vi "NavbalLabVIEW(15-5-28.vi"() -> ()   [LabVIEW 2012] (continued)
                }
              }
            }
          }
          "Phase Corner" <- w3618
          n781 = case "Pick out Mag, Phase, and Weight locations from Excel File" shown="True" "Slct Strt Pt" {
            tunnel: "Marker Listbox" -> [_ w3714]
            tunnel: w3337 -> [_ w3728]
            tunnel: w3329 -> [_ w3711]
            frame False {
            }
            frame True {
              n782 = property on="Marker Listbox" class="MCListbox (strict)"() -> ("ItemNames"=w3713:string[][])  [unwired: 2 in, 2 out]
              n783 = case shown="\"Stbd Side\"" w3711 {
                tunnel: [w3768 w3770] -> w3719
                tunnel: [4 ("y") 5 ("x")] -> w3708
                frame "Port Side", Default {
                  n784 = local read "#Stbd Accels"() -> (w3768:i32)
                }
                frame "Stbd Side" {
                  n785 = local read "#Port Accels"() -> (w3770:i32)
                }
              }
              n786 = Multiply(x=w3714, y=2) -> (x*y=w3726:i32)
              n787 = Increment(x=w3726) -> (x+1=w3724:i32)
              n788 = Index Array(array=w3713, index (row)=w3714, index (col)=0 ("disabled index (col)")) -> (element=→"Indicate Ref":string)
              n789 = call <vilib>:"New Report.vi"("report type"=T11."Excel", "template (empty)"=w3728) -> ("report out"=w3734:refnum<class "NI_report.lvclass">, "error out"=w3735:errorcluster)  [unwired: 12 in]
              n790 = Bundle("y"=12, w3724) -> (w3731:cluster{"y":i32, i32})  [unwired: 1 in]
              n791 = call <vilib>:"Excel Get Worksheet.vi"("report in"=w3734, "worksheet index (0)"=w3708, "error in (no error)"=w3735) -> ("report out"=w3737:refnum<class "NI_report.lvclass">, "error out"=w3738:errorcluster)  [unwired: 11 out]
              n792 = local read "#Corner Accels"() -> (w3718:i32)
              n793 = Increment(x=w3724) -> (x+1=w3725:i32)
              n794 = local read "#Corner Accels"() -> (w3709:i32)
              n795 = Add(x=w3718, y=w3719) -> (x+y=w3720:i32)
              n796 = Add(x=12, y=w3720) -> (x+y=w3722:i32)
              n797 = Decrement(x=w3722) -> (x-1=w3717:i32)
              n798 = Bundle(w3717, w3725) -> (w3730:cluster{i32, i32})  [unwired: 1 in]
              n799 = call-poly <vilib>:"Excel Get Data.vi"("report in"=w3737, "data type"=string[][] [], "start (-1, -1)"=w3731, "end (-1, -1)"=w3730, "error in (no error)"=w3738) -> ("data"=w3729:string[][], "error out"=w3723:errorcluster)  [unwired: 9 out]
              n800 = call <vilib>:"General Error Handler.vi"("error in (no error)"=w3723) -> ()  [unwired: 2 in, 13 out]
              n801 = Fract/Exp String To Number(string=w3729) -> (number=w3710:dbl[][])  [unwired: 3 in, 1 out]
              n802 = case shown="\"Port Side\", Default" w3711 {
                tunnel: w3710 -> [w3752 w3766]
                tunnel: [w3744 w3757] -> w3712
                tunnel: w3709 -> [w3741 w3756]
                frame "Port Side", Default {
                  n803 = Initialize Array(0.0 ("element"), w3741, 2 ("dimension size")) -> (w3749:dbl[][])
                  n804 = Insert Into Array(array=w3752, index (row)=0, new element=w3749) -> (w3748:dbl[][])  [unwired: 1 in]
                  n805 = Multiply(x=2, y=w3741) -> (x*y=w3740:i32)
                  n806 = local read "#Stbd Accels"() -> (w3739:i32)
                  n807 = Initialize Array(0.0 ("element"), w3739, 2 ("dimension size")) -> (w3745:dbl[][])
                  n808 = Insert Into Array(array=w3748, index (row)=w3740, new element=w3745) -> (w3744:dbl[][])  [unwired: 1 in]
                }
                frame "Stbd Side" {
                  n809 = local read "#Stbd Accels"() -> (w3753:i32)
                  n810 = Initialize Array(0.0 ("element"), w3756, 2 ("dimension size")) -> (w3763:dbl[][])
                  n811 = Insert Into Array(array=w3766, index (row)=w3756, new element=w3763) -> (w3762:dbl[][])  [unwired: 1 in]
                  n812 = Multiply(x=2, y=w3756) -> (x*y=w3754:i32)
                  n813 = Add(x=w3754, y=w3753) -> (x+y=w3761:i32)
                  n814 = Initialize Array(0.0 ("element"), w3753, 2 ("dimension size")) -> (w3758:dbl[][])
                  n815 = Insert Into Array(array=w3762, index (row)=w3761, new element=w3758) -> (w3757:dbl[][])  [unwired: 1 in]
                }
              }
              "Ref Pt Plot" <- w3712
            }
          }
          n816 = case shown="True" "Refresh Plot Listbox" {
            tunnel: w3337 -> [_ w3779]
            frame False {
            }
            frame True {
              n817 = local read "Port/Starboard"() -> (w3782:enum32{"Port Side", "Stbd Side"})
              n818 = case shown="\"Port Side\", Default" w3782 {
                tunnel: ["Data-Port" "Data-Stbd"] -> w3781
                frame "Port Side", Default {
                }
                frame "Stbd Side" {
                }
              }
              n819 = call <vilib>:"New Report.vi"("report type"=T11."Excel", "template (empty)"=w3779) -> ("report out"=w3785:refnum<class "NI_report.lvclass">, "error out"=w3784:errorcluster)  [unwired: 12 in]
              n820 = call <vilib>:"Excel Get Worksheet.vi"("report in"=w3785, "error in (no error)"=w3784, "name (\"\")"=w3781) -> ("report out"=w3798:refnum<class "NI_report.lvclass">, "error out"=w3797:errorcluster)  [unwired: 1 in, 10 out]
              n821 = Increment(x="# Runs") -> (x+1=w3786:dbl)
              n822 = Multiply(x=w3786, y=2) -> (x*y=w3788:dbl)
              n823 = Bundle("row"=2, w3788) -> (w3787:cluster{"row":i32, dbl})  [unwired: 1 in]
              n824 = call-poly <vilib>:"Excel Get Data.vi"("report in"=w3798, "data type"=string[][] [], "start (-1, -1)"=cluster{"row":i32, "column":i32} {"row"=0, "column"=1}, "end (-1, -1)"=w3787, "error in (no error)"=w3797) -> ("data"=w3792:string[][])  [unwired: 10 out]
              n825 = Transpose 2D Array(2D array=w3792) -> (transposed array=w3795:string[][])
              n826 = local read "Predicted Phase"() -> (w3775:dbl[])
              n827 = Index Array(array=w3795, index (col)=0 ("disabled index (col)")) -> (element=w3794:string[])  [unwired: 1 in]
              n828 = Decimate 1D Array(w3794) -> (w3791:string[])  [unwired: 1 out]
              n829 = Array Size(array=w3791) -> (size(s)=w3793:i32)
              n830 = Reshape Array(w3791, w3793, 1 ("dimension size")) -> (w3783:string[][])
              n831 = local read "Predicted Mag"() -> (w3776:dbl[])
              n832 = local read "Select Side to Analyze"() -> (w3771:enum32{"Starboard", "Port"})
              n833 = property on="Marker Listbox" class="MCListbox (strict)"("ItemNames"=w3783) -> ()  [unwired: 2 in, 2 out]
              n834 = local read "#Corner Accels"() -> (w3773:i32)
              n835 = Build Array(w3776, w3775) -> (w3777:dbl[][])
              n836 = Transpose 2D Array(2D array=w3777) -> (transposed array=w3774:dbl[][])
              n837 = case shown="\"Port\"" w3771 {
                tunnel: w3774 -> [w3815 w3829]
                tunnel: [w3806 w3821] -> w3772
                tunnel: w3773 -> [w3805 w3818]
                frame "Starboard", Default {
                  n838 = local read "#Stbd Accels"() -> (w3802:i32)
                  n839 = Initialize Array(0.0 ("element"), w3805, 2 ("dimension size")) -> (w3812:dbl[][])
                  n840 = Insert Into Array(array=w3815, index (row)=w3805, new element=w3812) -> (w3811:dbl[][])  [unwired: 1 in]
                  n841 = Multiply(x=2, y=w3805) -> (x*y=w3803:i32)
                  n842 = Add(x=w3803, y=w3802) -> (x+y=w3810:i32)
                  n843 = Initialize Array(0.0 ("element"), w3802, 2 ("dimension size")) -> (w3807:dbl[][])
                  n844 = Insert Into Array(array=w3811, index (row)=w3810, new element=w3807) -> (w3806:dbl[][])  [unwired: 1 in]
                }
                frame "Port" {
                  n845 = Initialize Array(0.0 ("element"), w3818, 2 ("dimension size")) -> (w3826:dbl[][])
                  n846 = Insert Into Array(array=w3829, index (row)=0, new element=w3826) -> (w3825:dbl[][])  [unwired: 1 in]
                  n847 = Multiply(x=2, y=w3818) -> (x*y=w3817:i32)
                  n848 = local read "#Stbd Accels"() -> (w3816:i32)
                  n849 = Initialize Array(0.0 ("element"), w3816, 2 ("dimension size")) -> (w3822:dbl[][])
                  n850 = Insert Into Array(array=w3825, index (row)=w3817, new element=w3822) -> (w3821:dbl[][])  [unwired: 1 in]
                }
              }
              "Pred plot" <- w3772
            }
          }
          n851 = Divide(x=159.0, y=w3556) -> (x/y=w3700:dbl)
          n852 = Divide(x=159.0, y=w3557) -> (x/y=w3685:dbl)
          n853 = Logarithm Base 10(1:w3700) -> (0:w3699:dbl)
          n854 = Divide(x=159.0, y=w3643) -> (x/y=w3658:dbl)
          n855 = Logarithm Base 10(1:w3685) -> (0:w3684:dbl)
          n856 = Divide(x=159.0, y=w3483) -> (x/y=w3509:dbl)
          n857 = Multiply(x=20.0, y=w3699) -> (x*y=w3698:dbl)
          n858 = Logarithm Base 10(1:w3658) -> (0:w3657:dbl)
          n859 = Multiply(x=20.0, y=w3684) -> (x*y=w3683:dbl)
          n860 = Logarithm Base 10(1:w3509) -> (0:w3508:dbl)
          n861 = Subtract(x=w3696, y=w3698) -> (x-y=w3692:dbl[][])
          "Magnitude AdB Stbd" <- w3692
          n862 = Multiply(x=20.0, y=w3657) -> (x*y=w3656:dbl)
          n863 = Subtract(x=w3681, y=w3683) -> (x-y=w3674:dbl[][])
          "Magnitude AdB Port" <- w3674
          n864 = Multiply(x=20.0, y=w3508) -> (x*y=w3507:dbl)
          n865 = Subtract(x=w3644, y=w3656) -> (x-y=w3642:dbl[][])
          "Magnitude AdB Corner" <- w3642
          n866 = Subtract(x=w3495, y=w3507) -> (x-y=w3494:dbl[][])
          "Magnitude AdB Corners-Port" <- w3494
          n867 = local read "Averaging"() -> (w3365:bool)
          n868 = for "Mils(8x)" {
            N: w3521 -> [_]
            tunnel: w3696 -> [w5013]
            tunnel: w3556 -> [w5009]
            tunnel: [w5008] -> w3639 mode=indexing
            tunnel: [w5007] -> w3697 mode=indexing
            i -> [w5010]
            n869 = Index Array(array=w5013, index (row)=w5010) -> (element=w5011:dbl[])  [unwired: 1 in]
            n870 = for {
              N: 8 -> [_]
              tunnel: w5011 -> [w5022]
              tunnel: w5009 -> [w5030]
              tunnel: [w5016] -> w5008 mode=indexing
              tunnel: [w5014] -> w5007 mode=indexing
              i -> [w5029]
              n871 = Add(x=w5029, y=1) -> (x+y=w5031:i32)
              n872 = Index Array(array=w5022, index=w5029) -> (element=w5023:dbl)
              n873 = Multiply(x=w5030, y=w5031) -> (x*y=w5014:dbl)
              n874 = Divide(x=159, y=w5014) -> (x/y=w5027:dbl)
              n875 = Logarithm Base 10(1:w5027) -> (0:w5026:dbl)
              n876 = Multiply(x=20.0, y=w5026) -> (x*y=w5024:dbl)
              n877 = Subtract(x=w5023, y=w5024) -> (x-y=w5017:dbl)
              n878 = Divide(x=w5017, y=20.0) -> (x/y=w5019:dbl)
              n879 = Power Of 10(x=w5019) -> (10^x=w5021:dbl)
              n880 = Multiply(x=w5021, y=0.0887) -> (x*y=w5015:dbl)
              n881 = Divide(x=w5015, y=w5014) -> (x/y=w5016:dbl)
            }
          }
          "Mils/sec Stbd" <- w3639
          "Freq Stbd" <- w3697
          n882 = for "Mils(8x)" {
            N: w3519 -> [_]
            tunnel: w3681 -> [w4905]
            tunnel: w3557 -> [w4901]
            tunnel: [w4900] -> w3619 mode=indexing
            tunnel: [w4899] -> w3682 mode=indexing
            i -> [w4902]
            n883 = Index Array(array=w4905, index (row)=w4902) -> (element=w4903:dbl[])  [unwired: 1 in]
            n884 = for {
              N: 8 -> [_]
              tunnel: w4903 -> [w4914]
              tunnel: w4901 -> [w4922]
              tunnel: [w4908] -> w4900 mode=indexing
              tunnel: [w4906] -> w4899 mode=indexing
              i -> [w4921]
              n885 = Add(x=w4921, y=1) -> (x+y=w4923:i32)
              n886 = Index Array(array=w4914, index=w4921) -> (element=w4915:dbl)
              n887 = Multiply(x=w4922, y=w4923) -> (x*y=w4906:dbl)
              n888 = Divide(x=159, y=w4906) -> (x/y=w4919:dbl)
              n889 = Logarithm Base 10(1:w4919) -> (0:w4918:dbl)
              n890 = Multiply(x=20.0, y=w4918) -> (x*y=w4916:dbl)
              n891 = Subtract(x=w4915, y=w4916) -> (x-y=w4909:dbl)
              n892 = Divide(x=w4909, y=20.0) -> (x/y=w4911:dbl)
              n893 = Power Of 10(x=w4911) -> (10^x=w4913:dbl)
              n894 = Multiply(x=w4913, y=0.0887) -> (x*y=w4907:dbl)
              n895 = Divide(x=w4907, y=w4906) -> (x/y=w4908:dbl)
            }
          }
          "Mils/sec Port" <- w3619
          "Freq Port" <- w3682
          n896 = Index Array(array=w3692, index (col)=0 ("disabled index (col)")) -> (element=w3693:dbl[])  [unwired: 1 in]
          n897 = local read "Averaging"() -> (w3358:bool)
          n898 = for "Mils(8x)" {
            N: w3571 -> [_]
            tunnel: w3644 -> [w4717]
            tunnel: w3643 -> [w4713]
            tunnel: [w4712] -> w3617 mode=indexing
            tunnel: [w4711] -> w3655 mode=indexing
            i -> [w4714]
            n899 = Index Array(array=w4717, index (row)=w4714) -> (element=w4715:dbl[])  [unwired: 1 in]
            n900 = for {
              N: 8 -> [_]
              tunnel: w4715 -> [w4726]
              tunnel: w4713 -> [w4734]
              tunnel: [w4720] -> w4712 mode=indexing
              tunnel: [w4718] -> w4711 mode=indexing
              i -> [w4733]
              n901 = Add(x=w4733, y=1) -> (x+y=w4735:i32)
              n902 = Index Array(array=w4726, index=w4733) -> (element=w4727:dbl)
              n903 = Multiply(x=w4734, y=w4735) -> (x*y=w4718:dbl)
              n904 = Divide(x=159, y=w4718) -> (x/y=w4731:dbl)
              n905 = Logarithm Base 10(1:w4731) -> (0:w4730:dbl)
              n906 = Multiply(x=20.0, y=w4730) -> (x*y=w4728:dbl)
              n907 = Subtract(x=w4727, y=w4728) -> (x-y=w4721:dbl)
              n908 = Divide(x=w4721, y=20.0) -> (x/y=w4723:dbl)
              n909 = Power Of 10(x=w4723) -> (10^x=w4725:dbl)
              n910 = Multiply(x=w4725, y=0.0887) -> (x*y=w4719:dbl)
              n911 = Divide(x=w4719, y=w4718) -> (x/y=w4720:dbl)
            }
          }
          "Mils/sec Corner" <- w3617
          "Freq Corner" <- w3655
          n912 = Index Array(array=w3674, index (col)=0 ("disabled index (col)")) -> (element=w3678:dbl[])  [unwired: 1 in]
          n913 = for "Mils(8x)" {
            N: w3481 -> [_]
            tunnel: w3495 -> [w4264]
            tunnel: w3483 -> [w4260]
            tunnel: [w4259] -> w3485 mode=indexing
            tunnel: [w4258] -> w3506 mode=indexing
            i -> [w4261]
            n914 = Index Array(array=w4264, index (row)=w4261) -> (element=w4262:dbl[])  [unwired: 1 in]
            n915 = for {
              N: 8 -> [_]
              tunnel: w4262 -> [w4273]
              tunnel: w4260 -> [w4281]
              tunnel: [w4267] -> w4259 mode=indexing
              tunnel: [w4265] -> w4258 mode=indexing
              i -> [w4280]
              n916 = Add(x=w4280, y=1) -> (x+y=w4282:i32)
              n917 = Index Array(array=w4273, index=w4280) -> (element=w4274:dbl)
              n918 = Multiply(x=w4281, y=w4282) -> (x*y=w4265:dbl)
              n919 = Divide(x=159, y=w4265) -> (x/y=w4278:dbl)
              n920 = Logarithm Base 10(1:w4278) -> (0:w4277:dbl)
              n921 = Multiply(x=20.0, y=w4277) -> (x*y=w4275:dbl)
              n922 = Subtract(x=w4274, y=w4275) -> (x-y=w4268:dbl)
              n923 = Divide(x=w4268, y=20.0) -> (x/y=w4270:dbl)
              n924 = Power Of 10(x=w4270) -> (10^x=w4272:dbl)
              n925 = Multiply(x=w4272, y=0.0887) -> (x*y=w4266:dbl)
              n926 = Divide(x=w4266, y=w4265) -> (x/y=w4267:dbl)
            }
          }
          "Mils/sec Corners-Port" <- w3485
          "Freq Corner Port" <- w3506
          n927 = local read "Averaging"() -> (w3356:bool)
          n928 = local read "Averaging"() -> (w3357:bool)
          n929 = Index Array(array=w3642, index (col)=0 ("disabled index (col)")) -> (element=w3652:dbl[])  [unwired: 1 in]
          n930 = Array Size(array=w3693) -> (size(s)=w3695:i32)
          n931 = Index Array(array=w3494, index (col)=0 ("disabled index (col)")) -> (element=w3503:dbl[])  [unwired: 1 in]
          n932 = Index Array(array=w3639, index (col)=0 ("index (row)")) -> (element=w3363:dbl[])  [unwired: 1 in]
          n933 = Index Array(array=w3558, index (col)=0 ("index")) -> (element=w3364:dbl[])  [unwired: 1 in]
          n934 = Index Array(array=w3692, index (col)=0 ("index (row)")) -> (element=w3361:dbl[])  [unwired: 1 in]
          n935 = Array Size(array=w3678) -> (size(s)=w3680:i32)
          n936 = Index Array(array=w3619, index (col)=0 ("index (row)")) -> (element=w3675:dbl[])  [unwired: 1 in]
          n937 = case shown="True" w3365 {
            tunnel: [w3879 w3880] -> w3362
            tunnel: w3364 -> [w3879 w3881]
            frame False {
            }
            frame True {
              n938 = call "Time Averaging3"("input signals"=w3881) -> ("time avg. signal"=w3880:dbl[])  [unwired: 15 in, 3 out]
            }
          }
          n939 = Index Array(array=w3415, index (col)=0 ("index")) -> (element=w3414:dbl[])  [unwired: 1 in]
          n940 = Index Array(array=w3674, index (col)=0 ("index (row)")) -> (element=w3673:dbl[])  [unwired: 1 in]
          n941 = Array Size(array=w3652) -> (size(s)=w3654:i32)
          n942 = for "Mils(1x)" {
            N: w3695 -> [_]
            tunnel: w3556 -> [w5002]
            tunnel: [w4997] -> w3360 mode=indexing
            tunnel: w3693 -> [w4996]
            i -> [w5006]
            n943 = Square(x=w5002) -> (x^2=w5000:dbl)
            n944 = Index Array(array=w4996, index #1=w5006) -> (element #1=w5005:dbl)  [unwired: 1 in, 1 out]
            n945 = Divide(x=0.028175, y=w5000) -> (x/y=w4998:dbl)
            n946 = Divide(x=w5005, y=20.0) -> (x/y=w5003:dbl)
            n947 = Power Of 10(x=w5003) -> (10^x=w4999:dbl)
            n948 = Multiply(x=w4999, y=w4998) -> (x*y=w4997:dbl)
          }
          "Mils(1x) Stbd" <- w3360
          n949 = case shown="True" w3358 {
            tunnel: w3414 -> [w3876 w3878]
            tunnel: [w3876 w3877] -> w3408
            frame False {
            }
            frame True {
              n950 = call "Time Averaging2"("input signals"=w3878) -> ("time avg. signal"=w3877:dbl[])  [unwired: 15 in, 3 out]
            }
          }
          n951 = Index Array(array=w3617, index (col)=0 ("index (row)")) -> (element=w3649:dbl[])  [unwired: 1 in]
          n952 = Index Array(array=w3618, index (col)=0 ("index")) -> (element=w3413:dbl[])  [unwired: 1 in]
          n953 = Index Array(array=w3642, index (col)=0 ("index (row)")) -> (element=w3648:dbl[])  [unwired: 1 in]
          n954 = Array Size(array=w3503) -> (size(s)=w3505:i32)
          n955 = for "Mils(1x)" {
            N: w3680 -> [_]
            tunnel: w3557 -> [w4894]
            tunnel: [w4889] -> w3677 mode=indexing
            tunnel: w3678 -> [w4888]
            i -> [w4898]
            n956 = Square(x=w4894) -> (x^2=w4892:dbl)
            n957 = Index Array(array=w4888, index #1=w4898) -> (element #1=w4897:dbl)  [unwired: 1 in, 1 out]
            n958 = Divide(x=0.028175, y=w4892) -> (x/y=w4890:dbl)
            n959 = Divide(x=w4897, y=20.0) -> (x/y=w4895:dbl)
            n960 = Power Of 10(x=w4895) -> (10^x=w4891:dbl)
            n961 = Multiply(x=w4891, y=w4890) -> (x*y=w4889:dbl)
          }
          "Mils(1x) Port" <- w3677
          n962 = Index Array(array=w3485, index (col)=0 ("index (row)")) -> (element=w3500:dbl[])  [unwired: 1 in]
          n963 = Index Array(array=w3486, index (col)=0 ("index")) -> (element=w3411:dbl[])  [unwired: 1 in]
          n964 = case shown="True" w3356 {
            tunnel: w3411 -> [w3870 w3872]
            tunnel: [w3870 w3871] -> w3410
            frame False {
            }
            frame True {
              n965 = call "Time Averaging5"("input signals"=w3872) -> ("time avg. signal"=w3871:dbl[])  [unwired: 15 in, 3 out]
            }
          }
          n966 = Index Array(array=w3494, index (col)=0 ("index (row)")) -> (element=w3499:dbl[])  [unwired: 1 in]
          n967 = case shown="True" w3357 {
            tunnel: w3413 -> [w3873 w3875]
            tunnel: [w3873 w3874] -> w3412
            frame False {
            }
            frame True {
              n968 = call "Time Averaging4"("input signals"=w3875) -> ("time avg. signal"=w3874:dbl[])  [unwired: 15 in, 3 out]
            }
          }
          n969 = for "Mils(1x)" {
            N: w3654 -> [_]
            tunnel: w3643 -> [w4706]
            tunnel: [w4701] -> w3651 mode=indexing
            tunnel: w3652 -> [w4700]
            i -> [w4710]
            n970 = Square(x=w4706) -> (x^2=w4704:dbl)
            n971 = Index Array(array=w4700, index #1=w4710) -> (element #1=w4709:dbl)  [unwired: 1 in, 1 out]
            n972 = Divide(x=0.028175, y=w4704) -> (x/y=w4702:dbl)
            n973 = Divide(x=w4709, y=20.0) -> (x/y=w4707:dbl)
            n974 = Power Of 10(x=w4707) -> (10^x=w4703:dbl)
            n975 = Multiply(x=w4703, y=w4702) -> (x*y=w4701:dbl)
          }
          "Mils(1x) Corners" <- w3651
          n976 = for "Mils(1x)" {
            N: w3505 -> [_]
            tunnel: w3483 -> [w4253]
            tunnel: [w4248] -> w3502 mode=indexing
            tunnel: w3503 -> [w4247]
            i -> [w4257]
            n977 = Square(x=w4253) -> (x^2=w4251:dbl)
            n978 = Index Array(array=w4247, index #1=w4257) -> (element #1=w4256:dbl)  [unwired: 1 in, 1 out]
            n979 = Divide(x=0.028175, y=w4251) -> (x/y=w4249:dbl)
            n980 = Divide(x=w4256, y=20.0) -> (x/y=w4254:dbl)
            n981 = Power Of 10(x=w4254) -> (10^x=w4250:dbl)
            n982 = Multiply(x=w4250, y=w4249) -> (x*y=w4248:dbl)
          }
          "Mils(1x) Corners-Port" <- w3502
          n983 = Build Array(w3363, w3362, w3361, w3360) -> (w3359:dbl[][])
          n984 = Build Array(w3675, w3408, w3673, w3677) -> (w3676:dbl[][])
          n985 = Build Array(w3649, w3412, w3648, w3651) -> (w3650:dbl[][])
          n986 = Build Array(w3500, w3410, w3499, w3502) -> (w3501:dbl[][])
          n987 = Transpose Matrix(1:w3359) -> (0:→"Starboard Arrays":dbl[][])
          n988 = Transpose Matrix(1:w3676) -> (0:→"Port Arrays":dbl[][])
          n989 = Transpose Matrix(1:w3650) -> (0:→"Corner Arrays Stbd":dbl[][])
          n990 = Transpose Matrix(1:w3501) -> (0:→"Corner Arrays Port":dbl[][])
          n991 = call <vilib>:"Value Has Changed PtByPt.vi"("input data point"=w3329) -> ("has changed"=w3341:bool)  [unwired: 1 in, 1 out]
          n992 = Or(x="Clear Save array", y=w3341) -> (x .or. y?=w3342:bool)
          n993 = Array Subset(array=w3639, index (col)=0 ("index"), length (col)=1 ("length")) -> (w3636:dbl[][])  [unwired: 2 in]
          n994 = Array Subset(array=w3558, index (col)=0 ("index"), length (col)=1 ("length")) -> (w3634:dbl[][])  [unwired: 2 in]
          n995 = case shown="True" w3342 {
            tunnel: w3329 -> [_ w3837]
            frame False {
            }
            frame True {
              n996 = local read "# of Runs to include"() -> (w3833:i32)
              n997 = local read "Boat File"() -> (w3840:path)
              n998 = case shown="\"Port Side\", Default" w3837 {
                tunnel: ["Data-Port" "Data-Stbd"] -> w3842
                frame "Port Side", Default {
                }
                frame "Stbd Side" {
                }
              }
              n999 = Multiply(x=w3833, y=2) -> (x*y=w3832:i32)
              n1000 = call <vilib>:"New Report.vi"("report type"=T11."Excel", "template (empty)"=w3840) -> ("report out"=w3844:refnum<class "NI_report.lvclass">, "error out"=w3843:errorcluster)  [unwired: 12 in]
              n1001 = call <vilib>:"Excel Get Worksheet.vi"("report in"=w3844, "error in (no error)"=w3843, "name (\"\")"=w3842) -> ("report out"=w3846:refnum<class "NI_report.lvclass">, "error out"=w3845:errorcluster)  [unwired: 1 in, 10 out]
              n1002 = Bundle("row"=0, w3832) -> (w3835:cluster{"row":i32, i32})  [unwired: 1 in]
              n1003 = call-poly <vilib>:"Excel Get Data.vi"("report in"=w3846, "data type"=string[][] [], "start (-1, -1)"=cluster{"row":i32, "column":i32} {"row"=0, "column"=1}, "end (-1, -1)"=w3835, "error in (no error)"=w3845) -> ("data"=w3848:string[][])  [unwired: 10 out]
              n1004 = Index Array(array=w3848, index (row)=0) -> (element=w3849:string[])  [unwired: 1 in]
              n1005 = Decimate 1D Array(w3849) -> (w3850:string[])  [unwired: 1 out]
              n1006 = local write "Weight+Location"(dbl[][] [[0.0, 0.0, 0.0, 0.0], [0.0, 0.0, 0.0, 0.0], [0.0, 0.0, 0.0, 0.0], [0.0, 0.0, 0.0, 0.0]] ("Weight+Location")) -> ()
              n1007 = property on="Run Reference:" class="Ring (strict)"("Strings []"=w3850) -> ()  [unwired: 2 in, 2 out]
            }
          }
          n1008 = Array Subset(array=w3617, index (col)=0 ("index"), length (col)=1 ("length")) -> (w3622:dbl[][])  [unwired: 2 in]
          n1009 = Array Subset(array=w3618, index (col)=0 ("index"), length (col)=1 ("length")) -> (w3620:dbl[][])  [unwired: 2 in]
          n1010 = Array Subset(array=w3485, index (col)=0 ("index"), length (col)=1 ("length")) -> (w3489:dbl[][])  [unwired: 2 in]
          n1011 = Insert Into Array(array=w3636, index (col)=1 ("disabled index (col)"), new element=w3634) -> (w3440:dbl[][])  [unwired: 1 in]
          "Mils/Sec-Phase(STBD)" <- w3440
          n1012 = Array Subset(array=w3486, index (col)=0 ("index"), length (col)=1 ("length")) -> (w3487:dbl[][])  [unwired: 2 in]
          n1013 = Insert Into Array(array=w3622, index (col)=1 ("disabled index (col)"), new element=w3620) -> (w3438:dbl[][])  [unwired: 1 in]
          "Mils/Sec-Phase(CORNERS-Stbd)" <- w3438
          n1014 = Insert Into Array(array=w3489, index (col)=1 ("disabled index (col)"), new element=w3487) -> (w3437:dbl[][])  [unwired: 1 in]
          "Mils/Sec-Phase(CORNERS-Port)" <- w3437
          n1015 = Array Subset(array=w3619, index (col)=0 ("index"), length (col)=1 ("length")) -> (w3629:dbl[][])  [unwired: 2 in]
          n1016 = Array Subset(array=w3415, index (col)=0 ("index"), length (col)=1 ("length")) -> (w3627:dbl[][])  [unwired: 2 in]
          n1017 = case shown="True" "Clear Strtpt" {
            frame False {
            }
            frame True {
              n1018 = local write "Ref Pt Plot"(dbl[][] [] ("Weight+Location")) -> ()
              n1019 = local write "Indicate Ref"("" ("Indicate Ref")) -> ()
            }
          }
          n1020 = Insert Into Array(array=w3629, index (col)=1 ("disabled index (col)"), new element=w3627) -> (w3439:dbl[][])  [unwired: 1 in]
          "Mils/Sec-Phase(PORT)" <- w3439
          n1021 = case "Saving run - Data Acquisition Tab" shown="True" "Save Run" {
            frame False {
            }
            frame True {
              w4629 = -4142 items=["xlRangeAutoFormat3DEffects1"=13, "xlRangeAutoFormat3DEffects2"=14, "xlRangeAutoFormatAccounting1"=4, "xlRangeAutoFormatAccounting2"=5, "xlRangeAutoFormatAccounting3"=6, "xlRangeAutoFormatAccounting4"=17, "xlRangeAutoFormatClassic1"=1, "xlRangeAutoFormatClassic2"=2, "xlRangeAutoFormatClassic3"=3, "xlRangeAutoFormatColor1"=7, "xlRangeAutoFormatColor2"=8, "xlRangeAutoFormatColor3"=9, "xlRangeAutoFormatList1"=10, "xlRangeAutoFormatList2"=11, "xlRangeAutoFormatList3"=12, "xlRangeAutoFormatLocalFormat1"=15, "xlRangeAutoFormatLocalFormat2"=16, "xlRangeAutoFormatLocalFormat3"=19, "xlRangeAutoFormatLocalFormat4"=20, "xlRangeAutoFormatReport1"=21, "xlRangeAutoFormatReport2"=22, "xlRangeAutoFormatReport3"=23, "xlRangeAutoFormatReport4"=24, "xlRangeAutoFormatReport5"=25, "xlRangeAutoFormatReport6"=26, "xlRangeAutoFormatReport7"=27, "xlRangeAutoFormatReport8"=28, "xlRangeAutoFormatReport9"=29, "xlRangeAutoFormatReport10"=30, "xlRangeAutoFormatClassicPivotTable"=31, "xlRangeAutoFormatTable1"=32, "xlRangeAutoFormatTable2"=33, "xlRangeAutoFormatTable3"=34, "xlRangeAutoFormatTable4"=35, "xlRangeAutoFormatTable5"=36, "xlRangeAutoFormatTable6"=37, "xlRangeAutoFormatTable7"=38, "xlRangeAutoFormatTable8"=39, "xlRangeAutoFormatTable9"=40, "xlRangeAutoFormatTable10"=41, "xlRangeAutoFormatPTNone"=42, "xlRangeAutoFormatNone"=-4142, "xlRangeAutoFormatSimple"=-4154] ("auto format (none)")
              w4618 = u16 3 items=["shift cells right", "shift cells down", "entire row", "entire column"] ("mode (entire row)")
              w4619 = cluster{"row":i32, "column":i32} {"row"=0, "column"=1} ("start (-1, -1)")
              w4547 = T18 {"font name"="Calibri", "font size"=12.0, "bold"=0, "italic"=0, "underline"=0, "strike through"=0, "font color"=0} ("font")
              # "4 planes"
              n1022 = local read "Divisions in\nEach Plane"() -> (w4588:T3)
              n1023 = Number To Fractional String(number="Weight+Location", precision (6)=i16 2) -> (F-format string=w4582:string[][])  [unwired: 2 in]
              n1024 = local read "time string"() -> (w4567:string)
              n1025 = Transpose 2D Array(2D array=w4582) -> (transposed array=w4577:string[][])
              n1026 = Index Array(array=w4588, index (col)=0 ("disabled index (col)")) -> (element=w4586:dbl[])  [unwired: 1 in]
              n1027 = for {
                N: 4 -> [_]
                tunnel: "Weight+Location" -> [w4693]
                tunnel: w4586 -> [w4671] mode=indexing
                tunnel: [w4659] -> w4585 mode=indexing
                tunnel: [w4657] -> w4584 mode=indexing
                i -> [w4692]
                n1028 = Index Array "Pick Plane"(array=w4693, index (row)=w4692) -> (element=w4687:dbl[])  [unwired: 1 in]
                n1029 = Index Array "Pick Mag"(array=w4687, index=0) -> (element=w4686:dbl)
                n1030 = Index Array "Pick Loc"(array=w4687, index=1) -> (element=w4685:dbl)
                n1031 = Index Array "Pick Mag"(array=w4687, index=2) -> (element=w4669:dbl)
                n1032 = Index Array "Pick Loc"(array=w4687, index=3) -> (element=w4672:dbl)
                n1033 = Decrement(x=w4685) -> (x-1=w4684:dbl)
                n1034 = Decrement(x=w4672) -> (x-1=w4673:dbl)
                n1035 = Divide(x=360.0, y=w4671) -> (x/y=w4651:dbl)
                n1036 = Multiply(x=w4651, y=w4684) -> (x*y=w4682:dbl)
                n1037 = Multiply(x=w4651, y=w4673) -> (x*y=w4674:dbl)
                n1038 = Multiply(x=w4682, y=3.141592653589793) -> (x*y=w4680:dbl)
                n1039 = Multiply(x=w4674, y=3.141592653589793) -> (x*y=w4676:dbl)
                n1040 = Divide(x=w4680, y=180.0) -> (x/y=w4678:dbl)
                n1041 = Divide(x=w4676, y=180.0) -> (x/y=w4670:dbl)
                n1042 = Polar To Complex(1:w4678, 2:w4686) -> (0:w4668:cdb)
                n1043 = Polar To Complex(1:w4670, 2:w4669) -> (0:w4667:cdb)
                n1044 = Add(x=w4668, y=w4667) -> (x+y=w4666:cdb)
                n1045 = Complex To Polar(r * e^(i*theta)=w4666) -> (r=w4658:dbl, theta=w4653:dbl)
                n1046 = Greater Or Equal To 0?(x=w4653) -> (x >= 0?=w4654:bool)
                n1047 = Add(x=w4653, y=6.283185307179586) -> (x+y=w4655:dbl)
                n1048 = Select(t=w4653, s=w4654, f=w4655) -> (s? t:f=w4652:dbl)
                n1049 = Multiply(x=w4652, y=180.0) -> (x*y=w4664:dbl)
                n1050 = Divide(x=w4664, y=3.141592653589793) -> (x/y=w4662:dbl)
                n1051 = Divide(x=w4662, y=w4651) -> (x/y=w4661:dbl)
                n1052 = Increment(x=w4661) -> (x+1=w4660:dbl)
                n1053 = Number To Fractional String(number=w4658) -> (F-format string=w4657:string)  [unwired: 3 in]
                n1054 = Number To Fractional String(number=w4660) -> (F-format string=w4659:string)  [unwired: 3 in]
              }
              n1055 = local read "date string"() -> (w4569:string)
              n1056 = Index Array(array=w4577, index (row)=0) -> (element=w4576:string[])  [unwired: 1 in]
              n1057 = Index Array(array=w4577, index (row)=1) -> (element=w4575:string[])  [unwired: 1 in]
              n1058 = Index Array(array=w4577, index (row)=2) -> (element=w4574:string[])  [unwired: 1 in]
              n1059 = Index Array(array=w4577, index (row)=3) -> (element=w4573:string[])  [unwired: 1 in]
              n1060 = for {
                tunnel: w4576 -> [w4631] mode=indexing
                tunnel: w4575 -> [w4633] mode=indexing
                tunnel: w4574 -> [w4635] mode=indexing
                tunnel: w4573 -> [w4638] mode=indexing
                tunnel: [w4640] -> w4572 mode=indexing
                tunnel: [w4639] -> w4571 mode=indexing
                n1061 = Equal?(x=w4631, y="0.00") -> (x = y?=w4632:bool)
                n1062 = Equal?(x=w4635, y="0.00") -> (x = y?=w4637:bool)
                n1063 = case shown="False" w4632 {
                  tunnel: w4631 -> [w4644 _]
                  tunnel: w4633 -> [w4643 _]
                  tunnel: [w4642 "" ("y")] -> w4640
                  frame False {
                    n1064 = Concatenate Strings(w4644, " @" ("string"), w4643) -> (w4642:string)
                  }
                  frame True {
                  }
                }
                n1065 = case shown="True" w4637 {
                  tunnel: w4635 -> [w4649 _]
                  tunnel: w4638 -> [w4648 _]
                  tunnel: [w4647 "" ("y")] -> w4639
                  frame False {
                    n1066 = Concatenate Strings(w4649, " @" ("string"), w4648) -> (w4647:string)
                  }
                  frame True {
                  }
                }
              }
              n1067 = Build Array("Save Run As:", w4569, w4567) -> (w4566:string[])
              n1068 = Build Array(w4572, w4571) -> (w4562:string[][])
              n1069 = Insert Into Array(array=string[][] [], index (row)=0, new element=w4566) -> (w4563:string[][])  [unwired: 1 in]
              n1070 = local read "Boat File"() -> (w4549:path)
              n1071 = Insert Into Array(array=w4562, index (col)=0 ("disabled index (col)"), new element=w4563) -> (w4550:string[][])  [unwired: 1 in]
              n1072 = case shown="\"Port Side\", Default" "Port/Starboard" {
                tunnel: ["Data-Port" "Data-Stbd"] -> w4595
                tunnel: ["Data-PortLog" ("name (\"\")") "Data-StbdLog" ("name (\"\")")] -> w4548
                frame "Port Side", Default {
                }
                frame "Stbd Side" {
                }
              }
              n1073 = Multiply(x="# of Runs to include", y=2) -> (x*y=w4532:i32)
              n1074 = call <vilib>:"New Report.vi"("report type"=T11."Excel", "template (empty)"=w4549) -> ("report out"=w4545:refnum<class "NI_report.lvclass">, "error out"=w4544:errorcluster)  [unwired: 12 in]
              n1075 = Bundle("row"=0, w4532) -> (w4533:cluster{"row":i32, i32})  [unwired: 1 in]
              n1076 = call <vilib>:"Excel Get Worksheet.vi"("report in"=w4545, "error in (no error)"=w4544, "name (\"\")"=w4595) -> ("report out"=w4539:refnum<class "NI_report.lvclass">, "error out"=w4538:errorcluster)  [unwired: 1 in, 10 out]
              n1077 = Array Size(array=w4585) -> (size(s)=w4609:i32)
              n1078 = call <vilib>:"Excel Get Worksheet.vi"("report in"=w4545, "error in (no error)"=w4544, "name (\"\")"=w4548) -> ("report out"=w4559:refnum<class "NI_report.lvclass">, "error out"=w4558:errorcluster)  [unwired: 1 in, 10 out]
              n1079 = call-poly <vilib>:"Excel Get Data.vi"("report in"=w4539, "data type"=string[][] [], "start (-1, -1)"=cluster{"row":i32, "column":i32} {"row"=0, "column"=1}, "end (-1, -1)"=w4533, "error in (no error)"=w4538) -> ("data"=w4543:string[][])  [unwired: 10 out]
              n1080 = call <vilib>:"Excel Get Last Row.vi"("report in"=w4559, "error in (no error)"=w4558) -> ("report out"=w4553:refnum<class "NI_report.lvclass">, "MS Office parameters out"=w4557:T14, "error out"=w4552:errorcluster)  [unwired: 11 in]
              n1081 = Reshape Array(w4585, w4609, 1 ("dimension size")) -> (w4608:string[][])
              n1082 = Unbundle(w4557) -> ("position (Excel)"=w4556:cluster{"row":i32, "column":i32})  [unwired: 2 out]
              n1083 = call <vilib>:"Excel Insert Cells.vi"("report in"=w4539, "mode (entire row)"=w4618, "start (0, 0)"=w4619, "error in (no error)"=w4538) -> ("report out"=w4621:refnum<class "NI_report.lvclass">, "error out"=w4620:errorcluster)  [unwired: 10 in]
              n1084 = Index Array(array=w4543, index (row)=0) -> (element=w4540:string[])  [unwired: 1 in]
              n1085 = Unbundle(w4556) -> ("row"=w4554:i32)  [unwired: 1 out]
              n1086 = call <vilib>:"Excel Insert Cells.vi"("report in"=w4621, "mode (entire row)"=w4618, "start (0, 0)"=w4619, "error in (no error)"=w4620) -> ("report out"=w4591:refnum<class "NI_report.lvclass">, "error out"=w4590:errorcluster)  [unwired: 10 in]
              n1087 = Decimate 1D Array(w4540) -> (w4536:string[])  [unwired: 1 out]
              n1088 = Index Array(array=w4536, index="Run Reference:") -> (element=w4535:string)
              n1089 = Build Array (concatenate)("Save Run As:", w4569, w4567, w4535, "Mag (mils/s)", w4584) -> (w4570:string[])
              n1090 = Array Size(array=w4570) -> (size(s)=w4607:i32)
              n1091 = Reshape Array(w4570, w4607, 1 ("dimension size")) -> (w4597:string[][])
              n1092 = Replace Array Subset(array=w4597, new element="Phase (deg)", index (row)=4 ("disabled index (col)"), index (col)=0 ("index")) -> (w4601:string[][])
              n1093 = Delete From Array(array=w4601, length=8, index (row)=5 ("disabled index (col)")) -> (array with subset deleted=w4600:string[][])  [unwired: 1 in, 1 out]
              n1094 = Build Array (concatenate)(w4600, w4608) -> (w4598:string[][])
              n1095 = Bundle("row"=w4554, "index"=0) -> (w4551:cluster{"row":i32, "index":i32})  [unwired: 1 in]
              n1096 = Insert Into Array(array=w4597, index (col)=1 ("disabled index (col)"), new element=w4598) -> (w4596:string[][])  [unwired: 1 in]
              "Excel Output Array" <- w4596
              n1097 = call-poly <vilib>:"Excel Easy Table.vi"("report in"=w4553, "font"=w4547, "start (0, 0)"=w4551, "text data"=w4550, "error in (no error)"=w4552) -> ()  [unwired: 6 in, 5 out]
              n1098 = call-poly <vilib>:"Excel Easy Table.vi"("report in"=w4591, "font"=w4547, "auto format (none)"=w4629, "start (0, 0)"=w4619, "text data"=w4596, "error in (no error)"=w4590) -> ("report out"=w4628:refnum<class "NI_report.lvclass">, "error out"=w4627:errorcluster)  [unwired: 5 in, 3 out]
              n1099 = case shown="\"Port Side\", Default" "Port/Starboard" {
                tunnel: [w4694 w4695] -> w4617
                frame "Port Side", Default {
                  n1100 = local read "Port Output Data"() -> (w4694:string[][])
                }
                frame "Stbd Side" {
                  n1101 = local read "Stbd Output Data"() -> (w4695:string[][])
                }
              }
              n1102 = Array Size(array=w4617) -> (size(s)=w4616:i32[])
              n1103 = Index Array(array=w4616, index=0) -> (element=w4614:i32)
              n1104 = Array Subset(array=w4617, index (row)=0 ("index"), length (row)=w4614, index (col)=1 ("length"), length (col)=2 ("length")) -> (w4594:string[][])
              n1105 = Array Subset(array=w4594) -> (w4592:string[][])  [unwired: 4 in]
              n1106 = call-poly <vilib>:"Excel Easy Table.vi"("report in"=w4628, "font"=w4547, "start (0, 0)"=cluster{"row":i32, "column":i32} {"row"=12, "column"=1} ("start (-1, -1)"), "text data"=w4592, "error in (no error)"=w4627) -> ("report out"=w4626:refnum<class "NI_report.lvclass">, "error out"=w4625:errorcluster)  [unwired: 6 in, 3 out]
              n1107 = call-dynamic "Save Report to File.vi"("report in"=w4626, "report file path"=w4549, "error in (no error)"=w4625) -> ()  [unwired: 11 in, 2 out]
            }
          }
          n1108 = Build Array (concatenate)(w3440, w3434) -> (w3474:dbl[][][])
          n1109 = Build Array (concatenate)(w3439, w3433) -> (w3344:dbl[][][])
          n1110 = Build Array (concatenate)(w3438, w3432) -> (w3473:dbl[][][])
          n1111 = Build Array (concatenate)(w3437, w3431) -> (w3472:dbl[][][])
          n1112 = for "Magnitude (AdB)" {
            N: w3571 -> [_]
            tunnel: w3480 -> [w4036]
            tunnel: [w4032] -> w3404 mode=indexing
            i -> [w4035]
            n1113 = Index Array(array=w4036, index=w4035) -> (element=w4030:cluster{"x0":dbl, "dx":dbl, "magnitude":dbl[]})
            n1114 = Unbundle(w4030) -> ("dx"=w4031:dbl, "magnitude"=w4033:dbl[])  [unwired: 1 out]
            n1115 = Array Size(array=w4033) -> (size(s)=w4034:i32)
            n1116 = for {
              N: w4034 -> [_]
              tunnel: w4031 -> [w4047]
              tunnel: w4033 -> [w4045]
              tunnel: [w4038] -> w4032 mode=indexing
              i -> [w4046]
              n1117 = Index Array(array=w4045, index=w4046) -> (element=w4037:dbl)
              n1118 = Multiply(x=w4047, y=w4046) -> (x*y=w4039:dbl)
              n1119 = Divide(x=159, y=w4039) -> (x/y=w4042:dbl)
              n1120 = Logarithm Base 10(1:w4042) -> (0:w4043:dbl)
              n1121 = Multiply(x=20.0, y=w4043) -> (x*y=w4040:dbl)
              n1122 = Subtract(x=w4037, y=w4040) -> (x-y=w4038:dbl)
            }
          }
          n1123 = for "Magnitude (AdB)" {
            N: w3521 -> [_]
            tunnel: w3478 -> [w4074]
            tunnel: [w4072] -> w3403 mode=indexing
            i -> [w4068]
            n1124 = Increment(x=w4068) -> (x+1=w4067:i32)
            n1125 = Index Array(array=w4074, index=w4067) -> (element=w4070:cluster{"x0":dbl, "dx":dbl, "magnitude":dbl[]})
            n1126 = Unbundle(w4070) -> ("dx"=w4071:dbl, "magnitude"=w4073:dbl[])  [unwired: 1 out]
            n1127 = Array Size(array=w4073) -> (size(s)=w4069:i32)
            n1128 = for {
              N: w4069 -> [_]
              tunnel: w4071 -> [w4085]
              tunnel: w4073 -> [w4083]
              tunnel: [w4076] -> w4072 mode=indexing
              i -> [w4084]
              n1129 = Index Array(array=w4083, index=w4084) -> (element=w4075:dbl)
              n1130 = Multiply(x=w4085, y=w4084) -> (x*y=w4077:dbl)
              n1131 = Divide(x=159, y=w4077) -> (x/y=w4080:dbl)
              n1132 = Logarithm Base 10(1:w4080) -> (0:w4081:dbl)
              n1133 = Multiply(x=20.0, y=w4081) -> (x*y=w4078:dbl)
              n1134 = Subtract(x=w4075, y=w4078) -> (x-y=w4076:dbl)
            }
          }
          n1135 = for "Magnitude (AdB)" {
            N: w3519 -> [_]
            tunnel: w3523 -> [w4055]
            tunnel: [w4053] -> w3402 mode=indexing
            i -> [w4049]
            n1136 = Increment(x=w4049) -> (x+1=w4048:i32)
            n1137 = Index Array(array=w4055, index=w4048) -> (element=w4051:cluster{"x0":dbl, "dx":dbl, "magnitude":dbl[]})
            n1138 = Unbundle(w4051) -> ("dx"=w4052:dbl, "magnitude"=w4050:dbl[])  [unwired: 1 out]
            n1139 = Array Size(array=w4050) -> (size(s)=w4054:i32)
            n1140 = for {
              N: w4054 -> [_]
              tunnel: w4052 -> [w4066]
              tunnel: w4050 -> [w4064]
              tunnel: [w4057] -> w4053 mode=indexing
              i -> [w4065]
              n1141 = Index Array(array=w4064, index=w4065) -> (element=w4056:dbl)
              n1142 = Multiply(x=w4066, y=w4065) -> (x*y=w4058:dbl)
              n1143 = Divide(x=159, y=w4058) -> (x/y=w4061:dbl)
              n1144 = Logarithm Base 10(1:w4061) -> (0:w4062:dbl)
              n1145 = Multiply(x=20.0, y=w4062) -> (x*y=w4059:dbl)
              n1146 = Subtract(x=w4056, y=w4059) -> (x-y=w4057:dbl)
            }
          }
          n1147 = property on="Tab 2" class="TabCtl (strict)"() -> ("Value"=w3454:T1)  [unwired: 2 in, 2 out]
          n1148 = property on="Tab 2" class="TabCtl (strict)"() -> ("Visible"=w3451:bool)  [unwired: 2 in, 2 out]
          n1149 = local read "#Corner Accels"() -> (w3373:i32)
          n1150 = local read "Sensor Info"() -> (w3471:string[][])
          n1151 = local read "#Stbd Accels"() -> (w3372:i32)
          n1152 = Less Or Equal?(x=w3454, y=T20."Step 4: Background Checks") -> (x <= y?=w3452:bool)
          n1153 = local read "#Port Accels"() -> (w3370:i32)
          n1154 = And(x=w3452, y=w3451) -> (x .and. y?=w3450:bool)
          n1155 = Index Array(array=w3478, index=0) -> (element=w3465:cluster{"x0":dbl, "dx":dbl, "magnitude":dbl[]})
          n1156 = Index Array(array=w3523, index=0) -> (element=w3469:cluster{"x0":dbl, "dx":dbl, "magnitude":dbl[]})
          n1157 = Index Array(array=w3480, index=0) -> (element=w3461:cluster{"x0":dbl, "dx":dbl, "magnitude":dbl[]})
          n1158 = Unbundle(w3465) -> ("x0"=w3464:dbl, "dx"=w3463:dbl)  [unwired: 1 out]
          n1159 = Unbundle(w3469) -> ("x0"=w3468:dbl, "dx"=w3467:dbl)  [unwired: 1 out]
          n1160 = Add(x=w3373, y=w3372) -> (x+y=w3371:i32)
          n1161 = Unbundle(w3461) -> ("x0"=w3460:dbl, "dx"=w3459:dbl)  [unwired: 1 out]
          n1162 = case shown="True" "Save Vibration Survey" {
            tunnel: w3404 -> [_ w3923]
            tunnel: w3403 -> [_ w3922]
            tunnel: w3402 -> [_ w3921]
            frame False {
            }
            frame True {
              w3917 = -4142 items=["xlRangeAutoFormat3DEffects1"=13, "xlRangeAutoFormat3DEffects2"=14, "xlRangeAutoFormatAccounting1"=4, "xlRangeAutoFormatAccounting2"=5, "xlRangeAutoFormatAccounting3"=6, "xlRangeAutoFormatAccounting4"=17, "xlRangeAutoFormatClassic1"=1, "xlRangeAutoFormatClassic2"=2, "xlRangeAutoFormatClassic3"=3, "xlRangeAutoFormatColor1"=7, "xlRangeAutoFormatColor2"=8, "xlRangeAutoFormatColor3"=9, "xlRangeAutoFormatList1"=10, "xlRangeAutoFormatList2"=11, "xlRangeAutoFormatList3"=12, "xlRangeAutoFormatLocalFormat1"=15, "xlRangeAutoFormatLocalFormat2"=16, "xlRangeAutoFormatLocalFormat3"=19, "xlRangeAutoFormatLocalFormat4"=20, "xlRangeAutoFormatReport1"=21, "xlRangeAutoFormatReport2"=22, "xlRangeAutoFormatReport3"=23, "xlRangeAutoFormatReport4"=24, "xlRangeAutoFormatReport5"=25, "xlRangeAutoFormatReport6"=26, "xlRangeAutoFormatReport7"=27, "xlRangeAutoFormatReport8"=28, "xlRangeAutoFormatReport9"=29, "xlRangeAutoFormatReport10"=30, "xlRangeAutoFormatClassicPivotTable"=31, "xlRangeAutoFormatTable1"=32, "xlRangeAutoFormatTable2"=33, "xlRangeAutoFormatTable3"=34, "xlRangeAutoFormatTable4"=35, "xlRangeAutoFormatTable5"=36, "xlRangeAutoFormatTable6"=37, "xlRangeAutoFormatTable7"=38, "xlRangeAutoFormatTable8"=39, "xlRangeAutoFormatTable9"=40, "xlRangeAutoFormatTable10"=41, "xlRangeAutoFormatPTNone"=42, "xlRangeAutoFormatNone"=-4142, "xlRangeAutoFormatSimple"=-4154] ("auto format (none)")
              w3893 = 1921 ("length")
              # "Collect from 10Hz - 490Hz\nThis will encompass 8 \nrotationals"
              n1163 = local read "Boat File"() -> (w3919:path)
              n1164 = Build Array (concatenate)(w3923, w3922, w3921) -> (w3920:dbl[][])
              n1165 = call <vilib>:"New Report.vi"("report type"=T11."Excel", "template (empty)"=w3919) -> ("report out"=w3905:refnum<class "NI_report.lvclass">, "error out"=w3904:errorcluster)  [unwired: 12 in]
              n1166 = call <vilib>:"Excel Add Worksheet.vi"("report in"=w3905, "error in (no error)"=w3904) -> ("report out"=w3903:refnum<class "NI_report.lvclass">, "error out"=w3902:errorcluster)  [unwired: 12 in]
              n1167 = Transpose 2D Array(2D array=w3920) -> (transposed array=w3927:dbl[][])
              n1168 = call <vilib>:"Excel Workbook Properties.vi"("report in"=w3903, "error in (no error)"=w3902) -> ("report out"=w3912:refnum<class "NI_report.lvclass">, "worksheets count"=w3901:i32, "error out"=w3911:errorcluster)  [unwired: 10 in, 1 out]
              n1169 = Decrement(x=w3901) -> (x-1=w3900:i32)
              n1170 = Array Subset(array=w3927, index (row)=40 ("index"), length (row)=w3893) -> (w3924:dbl[][])  [unwired: 2 in]
              n1171 = for {
                N: w3893 -> [_]
                tunnel: [w3928] -> w3891 mode=indexing
                i -> [w3934]
                n1172 = Multiply(x=0.25, y=w3934) -> (x*y=w3932:dbl)
                n1173 = Add(x=10.0, y=w3932) -> (x+y=w3929:dbl)
                n1174 = Number To Fractional String(number=w3929, precision (6)=i16 3 ("width (-)")) -> (F-format string=w3928:string)  [unwired: 2 in]
              }
              n1175 = call <vilib>:"Excel Get Worksheet.vi"("report in"=w3912, "worksheet index (0)"=w3900, "error in (no error)"=w3911) -> ("report out"=w3910:refnum<class "NI_report.lvclass">, "error out"=w3909:errorcluster)  [unwired: 11 out]
              n1176 = call <vilib>:"Excel Rename Worksheet.vi"("report in"=w3910, "worksheet name (\"\")"="Vibration Survey Name", "error in (no error)"=w3909) -> ("report out"=w3908:refnum<class "NI_report.lvclass">, "error out"=w3907:errorcluster)  [unwired: 11 in]
              n1177 = Number To Fractional String(number=w3924, precision (6)=i16 3 ("width (-)")) -> (F-format string=w3884:string[][])  [unwired: 2 in]
              n1178 = Insert Into Array(array=w3884, index (col)=0 ("disabled index (col)"), new element=w3891) -> (w3883:string[][])  [unwired: 1 in]
              n1179 = local read "# Accel Channels"() -> (w3897:i32)
              n1180 = local read "Sensor Info"() -> (w3899:string[][])
              n1181 = Array Subset(array=w3899, index (row)=0 ("index"), length (row)=w3897, index (col)=0 ("index"), length (col)=1 ("length")) -> (w3890:string[][])
              n1182 = Index Array(array=w3890, index (col)=0 ("disabled index (col)")) -> (element=w3888:string[])  [unwired: 1 in]
              n1183 = Insert Into Array(array=w3888, index=0, new element=" " ("new element/subarray")) -> (w3885:string[])
              n1184 = Insert Into Array(array=w3883, index (row)=0, new element=w3885) -> (w3882:string[][])  [unwired: 1 in]
              n1185 = call-poly <vilib>:"Excel Easy Table.vi"("report in"=w3908, "font"=T18 {"font name"="Calibri", "font size"=12.0, "bold"=0, "italic"=0, "underline"=0, "strike through"=0, "font color"=0}, "auto format (none)"=w3917, "start (0, 0)"=cluster{"row":i32, "column":i32} {"row"=0, "column"=0}, "text data"=w3882, "error in (no error)"=w3907) -> ("report out"=w3915:refnum<class "NI_report.lvclass">, "error out"=w3914:errorcluster)  [unwired: 5 in, 3 out]
              n1186 = call-dynamic "Save Report to File.vi"("report in"=w3915, "report file path"=w3919, "error in (no error)"=w3914) -> ()  [unwired: 11 in, 2 out]
            }
          }
          n1187 = local read "Corner Arrays Stbd"() -> (w3377:dbl[][])
          n1188 = local read "Corner Arrays Port"() -> (w3376:dbl[][])
          n1189 = local read "Starboard Arrays"() -> (w3375:dbl[][])
          n1190 = Bundle("x0"=w3464, "dx"=w3463, w3403) -> (w3400:cluster{"x0":dbl, "dx":dbl, dbl[][]})  [unwired: 1 in]
          n1191 = Bundle("x0"=w3468, "dx"=w3467, w3402) -> (w3399:cluster{"x0":dbl, "dx":dbl, dbl[][]})  [unwired: 1 in]
          n1192 = local read "Port Arrays"() -> (w3374:dbl[][])
          n1193 = Bundle("x0"=w3460, "dx"=w3459, w3404) -> (w3458:cluster{"x0":dbl, "dx":dbl, dbl[][]})  [unwired: 1 in]
          n1194 = Array Subset(array=w3471, index (row)=0 ("index"), length (row)=w3373, index (col)=0 ("index"), length (col)=1 ("length")) -> (w3348:string[][])
          n1195 = Array Subset(array=w3471, index (row)=w3373, length (row)=w3372, index (col)=0 ("index"), length (col)=1 ("length")) -> (w3378:string[][])
          n1196 = Array Subset(array=w3471, index (row)=w3371, length (row)=w3370, index (col)=0 ("index"), length (col)=1 ("length")) -> (w3384:string[][])
          n1197 = for {
            tunnel: w3348 -> [w3860] mode=indexing
            tunnel: [w3859] -> w3354 mode=indexing
            n1198 = for {
              tunnel: w3860 -> [w3863] mode=indexing
              tunnel: [w3861] -> w3859 mode=indexing
              n1199 = Concatenate Strings(w3863, "-S" ("string")) -> (w3861:string)
            }
          }
          n1200 = Number To Fractional String(number=w3377, precision (6)=i16 3 ("width (-)")) -> (F-format string=w3396:string[][])  [unwired: 2 in]
          n1201 = Number To Fractional String(number=w3376, precision (6)=i16 3 ("width (-)")) -> (F-format string=w3393:string[][])  [unwired: 2 in]
          n1202 = Build Array (concatenate)(w3404, w3404, w3403, w3402) -> (w3405:dbl[][])
          n1203 = Number To Fractional String(number=w3375, precision (6)=i16 3 ("width (-)")) -> (F-format string=w3390:string[][])  [unwired: 2 in]
          n1204 = Number To Fractional String(number=w3374, precision (6)=i16 3 ("width (-)")) -> (F-format string=w3381:string[][])  [unwired: 2 in]
          n1205 = for {
            tunnel: [w3855] -> w3349 mode=indexing
            tunnel: w3348 -> [w3854] mode=indexing
            n1206 = for {
              tunnel: [w3857] -> w3855 mode=indexing
              tunnel: w3854 -> [w3856] mode=indexing
              n1207 = Concatenate Strings(w3856, "-P" ("string")) -> (w3857:string)
            }
          }
          n1208 = case shown="True" w3450 {
            tunnel: w3666 -> [_ w4029]
            tunnel: w3665 -> [_ w4028]
            tunnel: w3477 -> [_ w4027]
            tunnel: w3399 -> [_ w4026]
            tunnel: w3400 -> [_ w4025]
            tunnel: w3458 -> [_ w4024]
            tunnel: w3457 -> [_ w4023]
            tunnel: w3456 -> [_ w4022]
            frame False {
            }
            frame True {
              # "Sensor Overview"
              "AdB Port" <- w4026
              "AdB Starboard" <- w4025
              "Tach Signal Port" <- w4029
              "Accelerometer Signals Port" <- w4028
              "Tach Signal Stbd" <- w4027
              "Accelerometer Signals Stbd" <- w4023
              "AdB Corners" <- w4024
              "Accelerometer Signals Corners" <- w4022
            }
          }
          n1209 = Array Size(array="MagPhase") -> (size(s)=w3561:i32)
          n1210 = Insert Into Array(array=w3349, index (col)=1 ("disabled index (col)"), new element=w3393) -> (w3346:string[][])  [unwired: 1 in]
          n1211 = Insert Into Array(array=w3354, index (col)=1 ("disabled index (col)"), new element=w3396) -> (w3352:string[][])  [unwired: 1 in]
          n1212 = Insert Into Array(array=w3378, index (col)=1 ("disabled index (col)"), new element=w3390) -> (w3351:string[][])  [unwired: 1 in]
          n1213 = Insert Into Array(array=w3384, index (col)=1 ("disabled index (col)"), new element=w3381) -> (w3345:string[][])  [unwired: 1 in]
          n1214 = for {
            N: w3561 -> [_]
            tunnel: "MagPhase" -> [w4524]
            tunnel: w3405 -> [w4525]
            tunnel: [w4520] -> w3560 mode=indexing
            tunnel: u32[] [4342527, 16728642, 3079936, 46079, 16776704, 14768639, 16753962, 6399, 16728757, 5896447, 0, 16777215, 16711422, 16777215, 16777215, 16777215, 16448250, 16711422, 16777215] -> [w4521] mode=indexing
            i -> [w4523]
            n1215 = flat-sequence {
              tunnel: w4522 -> [w4527]
              tunnel: w4521 -> [w4529]
              frame #0 {
                n1216 = Bundle(w4527, 5) -> (w4526:cluster{i32, i32})  [unwired: 1 in]
                n1217 = property on="MagPhase" class="MCListbox (strict)"("ActiveCell"=w4526) -> ()  [unwired: 2 in, 2 out]
              }
              frame #1 {
                n1218 = property on="MagPhase" class="MCListbox (strict)"("CellBG"=w4529) -> ()  [unwired: 2 in, 2 out]
              }
            }
            n1219 = Index Array(array=w4524, index=w4523) -> (element=w4522:i32)
            n1220 = Index Array(array=w4525, index (row)=w4522) -> (element=w4520:dbl[])  [unwired: 1 in]
          }
          n1221 = Build Array (concatenate)(w3352, w3346, w3351, w3345) -> (w3398:string[][])
          n1222 = Build Array (concatenate)(w3352, w3351) -> (→"Stbd Output Data":string[][])
          n1223 = Build Array (concatenate)(w3346, w3345) -> (→"Port Output Data":string[][])
          n1224 = Index Array(array=w3478, index=0) -> (element=w3565:cluster{"x0":dbl, "dx":dbl, "magnitude":dbl[]})
          n1225 = Unbundle(w3565) -> ("x0"=w3564:dbl, "dx"=w3563:dbl)  [unwired: 1 out]
          n1226 = property on="MagPhase" class="MCListbox (strict)"("ItemNames"=w3398) -> ()  [unwired: 2 in, 2 out]
          n1227 = property on="DAQ Listbox" class="MCListbox (strict)"("ItemNames"=w3398) -> ()  [unwired: 2 in, 2 out]
          n1228 = Bundle("x0"=w3564, "dx"=w3563, w3560) -> (→"Spectrum (AdB)":cluster{"x0":dbl, "dx":dbl, dbl[][]})  [unwired: 1 in]
        }
      }
    }
    n1229 = case "Accelerometer Calibration" shown="True" "Accel Calib Start" {
      tunnel: w366 -> [w3145 _]
      tunnel: "Ship Class" -> [_ w3147]
      frame False {
        n1230 = call-poly <userlib>:"Circular Buffer.vi"("Buffer Size"=w3145, "Operation"=Circular_Buffer_Operations."Initialize") -> ()  [unwired: 6 in, 4 out]
        n1231 = property on="DAQ Start" class="Bool (strict)"("DisabledEnum"=T16."Enabled" ("Disabled")) -> ()  [unwired: 2 in, 2 out]
      }
      frame True {
        # "Enter in the channel list from the excel sheet"
        # "Initialize buffer variable\n1024 samples per channel\n# accelerometer channels"
        # "ignore the first 12 rows because\nthey are the repeated corner accels"
        n1232 = local read "# Accel Channels"() -> (w3148:i32)
        n1233 = local read "# Accel Channels"() -> (w3152:i32)
        n1234 = local read "Sensor Info"() -> (w3161:string[][])
        n1235 = Bundle("Samples per Channel"=u32 1024, "# Accel Channels"=w3148) -> (w3149:T24)  [unwired: 1 in]
        n1236 = while "Write into buffer variable" {
          tunnel: w3149 -> [w3165]
          tunnel: w3147 -> [w3162]
          stop <- w3164 stop-if-true
          n1237 = local read "Accel Calib Start"() -> (w3163:bool)
          n1238 = Not(x=w3163) -> (.not. x?=w3164:bool)
          n1239 = case shown="\"LA Class\"" w3162 {
            tunnel: [w3169 w3170 w3173] -> w3166
            tunnel: w3164 -> [w3168 w3171 w3172]
            frame "Simulated Signals Ohio", Default {
              n1240 = call "DAQ Assistant Accel Calib Ohio2"("stop (F)"=w3168) -> ("data"=w3169:dynamicdata)  [unwired: 15 in, 3 out]
            }
            frame "LA Class" {
              n1241 = call "DAQ Assistant Accel Calib LAclass"("stop (F)"=w3171) -> ("data"=w3170:dynamicdata)  [unwired: 15 in, 3 out]
            }
            frame "Ohio Class" {
              n1242 = call "DAQ Assistant Accel Calib Ohio"("stop (F)"=w3172) -> ("data"=w3173:dynamicdata)  [unwired: 15 in, 3 out]
            }
          }
          n1243 = call-poly <userlib>:"Circular Buffer.vi"("Buffer Size"=w3165, "Operation"=Circular_Buffer_Operations."Write", "Data In"=w3166) -> ()  [unwired: 5 in, 4 out]
        }
        n1244 = call-poly <userlib>:"Circular Buffer.vi"("Buffer Size"=w3149, "Operation"=Circular_Buffer_Operations."Initialize") -> ()  [unwired: 6 in, 4 out]
        n1245 = Array Subset(array=w3161, index (row)=0 ("index"), length (row)=w3152, index (col)=0 ("index"), length (col)=2 ("length")) -> (w3151:string[][])
        n1246 = Insert Into Array(array=w3151, index (col)=2 ("disabled index (col)"), new element=string[] ["", "", "", "", "", "", "", "", "", "", "", "", "", "", "", "", "", "", "", "", "", "", "", "", "", "", "", "", "", "", " ", "", "", "", "", "", "", "", "", "", ""] ("new element/subarray")) -> (w3160:string[][])  [unwired: 1 in]
        n1247 = property on="DAQ Start" class="Bool (strict)"("DisabledEnum"=T16."Disabled and Grayed Out" ("Disabled")) -> ()  [unwired: 2 in, 2 out]
        n1248 = property on="Calibration Channel List" class="MCListbox (strict)"("ItemNames"=w3160) -> ()  [unwired: 2 in, 2 out]
        n1249 = while "Read from buffer, Write calibration values" {
          tunnel: w3149 -> [w3177]
          stop <- w3184 stop-if-true
          n1250 = Unbundle(w3177) -> ("Samples per Channel"=w3176:u32)  [unwired: 1 out]
          n1251 = local read "Accel Calib Start"() -> (w3175:bool)
          n1252 = Not(x=w3175) -> (.not. x?=w3184:bool)
          n1253 = call-poly <userlib>:"Circular Buffer.vi"("Buffer Size"=w3177, "Read Size"=w3176, "Operation"=Circular_Buffer_Operations."Read (most recent)") -> ("Data Out"=w3174:waveform(dbl)[])  [unwired: 5 in, 3 out]
          n1254 = call "Convert from Dynamic Data3"("Dynamic Data Type"=w3174) -> ("Array"=w3179:dbl[][])  [unwired: 3 in]
          n1255 = Array Size(array=w3179) -> (size(s)=w3182:i32[])
